vi "KGN Get actual Values 1.vi"(7 "scaling":dbl, 8 "Fehler (Eingang, kein Fehler)":errorcluster, 9 "Info Cluster":T1, 10 "VISA-Referenz (Eingang)":refnum<visa-resource-name>, 11 "device (Eingang)":u32) -> (0 "Fehler (Ausgang)":errorcluster, 1 "Info Cluster out":T1, 2 "VISA-Referenz (Ausgang)":refnum<visa-resource-name>, 3 "dup device (Ausgang)":u32, 4 "actual Values Cluster":T4 {"Cluster"."PumpModeGeneral-Cluster"."dry mode" items=["wet", "dry"]; "Cluster"."PumpModeGeneral-Cluster"."control mode" items=["static", "pid"]}, 5 "Kommandos gesendet":string, 6 "connected":bool)   [LabVIEW 2020, in "Linearisierung v2.lvlib" / "Gasteiler.lvlib" / "HovaCAL_Interface.lvlib" / "KGN.lvlib" / "KGN GUI Get.lvlib"]
uses:
  KGN GUI Get.lvlib
  Controls/Info Cluster.ctl
  Controls/Pump Dry Mode.ctl
  Controls/Pump Control Mode.ctl
  Controls/Controls.lvlib
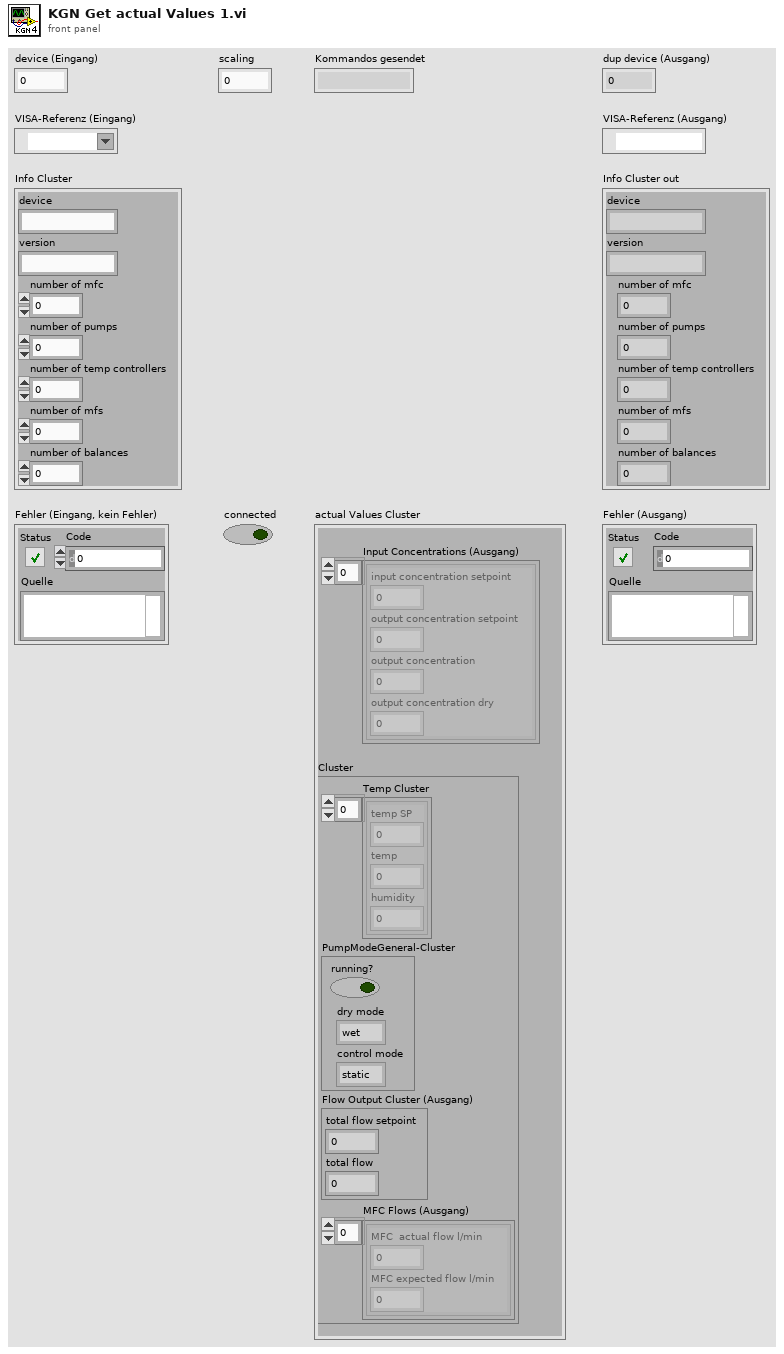
[diagram p1: front panel]
types:
  T1 = typedef "Linearisierung v2.lvlib/Gasteiler.lvlib/HovaCAL_Interface.lvlib/Controls.lvlib/Info Cluster.ctl" = cluster{"device":string, "version":string, "number of mfc":i32, "number of pumps":i32, "number of temp controllers":i32, "number of mfs":i32, "number of balances":i32}
  T2 = typedef "Linearisierung v2.lvlib/Gasteiler.lvlib/HovaCAL_Interface.lvlib/Controls.lvlib/Pump Dry Mode.ctl" = i32
  T3 = typedef "Linearisierung v2.lvlib/Gasteiler.lvlib/HovaCAL_Interface.lvlib/Controls.lvlib/Pump Control Mode.ctl" = u32
  T4 = cluster{"Input Concentrations (Ausgang)":cluster{"input concentration setpoint":dbl, "output concentration setpoint":dbl, "output concentration":dbl, "output concentration dry":dbl}[], "Cluster":cluster{"Temp Cluster":cluster{"temp SP":dbl, "temp":dbl, "humidity":dbl}[], "PumpModeGeneral-Cluster":cluster{"running?":bool, "dry mode":T2, "control mode":T3}, "Flow Output Cluster (Ausgang)":cluster{"total flow setpoint":dbl, "total flow":dbl}, "MFC Flows (Ausgang)":cluster{"MFC  actual flow l/min":dbl, "MFC expected flow l/min":dbl}[]}}
  T5 = cluster{"input concentration setpoint":dbl, "output concentration setpoint":dbl, "output concentration":dbl, "output concentration dry":dbl}[]
  T6 = cluster{"temp SP":dbl, "temp":dbl, "humidity":dbl}[]
  T7 = cluster{"running?":bool, "dry mode":T2, "control mode":T3}
  T8 = cluster{"total flow setpoint":dbl, "total flow":dbl}
  T9 = cluster{"MFC  actual flow l/min":dbl, "MFC expected flow l/min":dbl}[]
  T10 = cluster{"Temp Cluster":cluster{"temp SP":dbl, "temp":dbl, "humidity":dbl}[], "PumpModeGeneral-Cluster":cluster{"running?":bool, "dry mode":T2, "control mode":T3}, "Flow Output Cluster (Ausgang)":cluster{"total flow setpoint":dbl, "total flow":dbl}, "MFC Flows (Ausgang)":cluster{"MFC  actual flow l/min":dbl, "MFC expected flow l/min":dbl}[]}
  T11 = cluster{"Input Concentrations (Ausgang)":cluster{"input concentration setpoint":dbl, "output concentration setpoint":dbl, "output concentration":dbl, "output concentration dry":dbl}[], cluster{"Temp Cluster":cluster{"temp SP":dbl, "temp":dbl, "humidity":dbl}[], "PumpModeGeneral-Cluster":cluster{"running?":bool, "dry mode":T2, "control mode":T3}, "Flow Output Cluster (Ausgang)":cluster{"total flow setpoint":dbl, "total flow":dbl}, "MFC Flows (Ausgang)":cluster{"MFC  actual flow l/min":dbl, "MFC expected flow l/min":dbl}[]}}
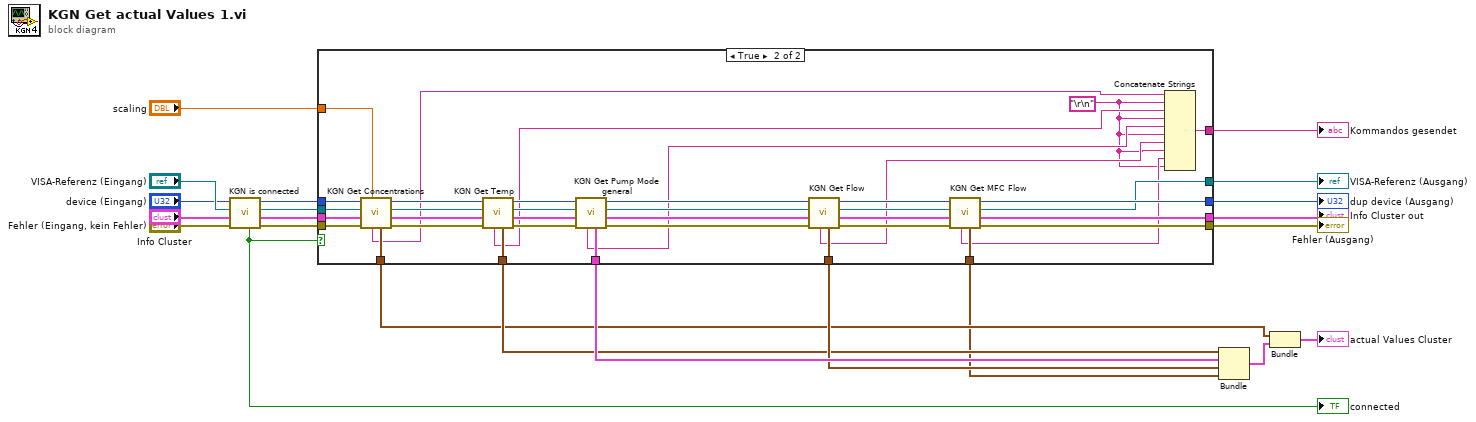
[diagram p0: block diagram]
diagram:
  n1 = call "KGN is connected.vi"("VISA-Ressourcenname"="VISA-Referenz (Eingang)", "device"="device (Eingang)") -> ("VISA-Ressourcenname out"=w19:refnum<visa-resource-name>, "dup device out"=w18:u32, "Boolesch"=w17:bool)  [unwired: 6 in, 1 out]
  "connected" <- w17
  n2 = case shown="True" w17 {
    tunnel: "Fehler (Eingang, kein Fehler)" -> [w24 w61]
    tunnel: [w24 w33] -> w8
    tunnel: w18 -> [w23 w60]
    tunnel: [_ w51] -> w6
    tunnel: "Info Cluster" -> [w21 w53]
    tunnel: [w23 w39] -> w9
    tunnel: "scaling" -> [_ w42]
    tunnel: [_ w48] -> w11
    tunnel: [_ w41] -> w12
    tunnel: [_ w45] -> w13
    tunnel: w19 -> [w22 w52]
    tunnel: [w22 w37] -> w20
    tunnel: [w21 w35] -> w4
    tunnel: [_ w32] -> w2
    tunnel: [_ w25] -> w1
    frame False {
    }
    frame True {
      w26 = "\r\n"
      n3 = call "KGN Get Concentrations.vi"("scaling"=w42, "Fehler (Eingang, kein Fehler)"=w61, "Info Cluster"=w53, "VISA-Ressourcenname"=w52, "device (Eingang)"=w60) -> ("Fehler (Ausgang)"=w59:errorcluster, "Info Cluster out"=w50:T1, "VISA-Ressourcenname out"=w49:refnum<visa-resource-name>, "dup device (Ausgang)"=w58:u32, "Input Concentrations (Ausgang)"=w51:T5, "Kommandos gesendet"=w31:string)  [unwired: 1 in]
      n4 = call "KGN Get Temp.vi"("Fehler (Eingang, kein Fehler)"=w59, "Info Cluster"=w50, "VISA-Ressourcenname"=w49, "device (Eingang)"=w58) -> ("Fehler (Ausgang)"=w57:errorcluster, "Info Cluster out"=w46:T1, "VISA-Ressourcenname out"=w47:refnum<visa-resource-name>, "dup device (Ausgang)"=w55:u32, "Temp Cluster"=w48:T6, "Kommandos gesendet"=w30:string)  [unwired: 2 in]
      n5 = call "KGN Get Pump Mode general.vi"("Fehler (Eingang, kein Fehler)"=w57, "Info Cluster"=w46, "VISA-Ressourcenname"=w47, "device (Eingang)"=w55) -> ("Fehler (Ausgang)"=w56:errorcluster, "Info Cluster out"=w44:T1, "VISA-Ressourcenname out"=w43:refnum<visa-resource-name>, "dup device (Ausgang)"=w54:u32, "PumpModeGeneral-Cluster"=w45:T7, "Kommandos gesendet"=w29:string)  [unwired: 2 in]
      n6 = call "KGN Get Flow.vi"("Fehler (Eingang, kein Fehler)"=w56, "Info Cluster"=w44, "VISA-Referenz (Eingang)"=w43, "device (Eingang)"=w54) -> ("Fehler (Ausgang)"=w34:errorcluster, "Info Cluster out"=w36:T1, "VISA-Referenz (Ausgang)"=w38:refnum<visa-resource-name>, "dup device"=w40:u32, "Flow Output Cluster (Ausgang)"=w41:T8, "Kkommandos gesendet"=w28:string)  [unwired: 2 in]
      n7 = call "KGN Get MFC Flow.vi"("Fehler (Eingang, kein Fehler)"=w34, "Info Cluster"=w36, "VISA-Ressourcenname"=w38, "device (Eingang)"=w40) -> ("Fehler (Ausgang)"=w33:errorcluster, "Info Cluster out"=w35:T1, "VISA-Ressourcenname out"=w37:refnum<visa-resource-name>, "dup device (Ausgang)"=w39:u32, "MFC Flows (Ausgang)"=w32:T9, "Kommandos gesendet"=w27:string)  [unwired: 2 in]
      n8 = Concatenate Strings(w31, w26, w30, w26, w29, w26, w28, w26, w27, w26) -> (w25:string)
    }
  }
  "VISA-Referenz (Ausgang)" <- w20
  "dup device (Ausgang)" <- w9
  "Fehler (Ausgang)" <- w8
  "Info Cluster out" <- w4
  "Kommandos gesendet" <- w1
  n9 = Bundle("Temp Cluster"=w11, "PumpModeGeneral-Cluster"=w13, "Flow Output Cluster (Ausgang)"=w12, "MFC Flows (Ausgang)"=w2) -> (w5:T10)  [unwired: 1 in]
  n10 = Bundle("Input Concentrations (Ausgang)"=w6, w5) -> (→"actual Values Cluster":T11)  [unwired: 1 in]
